vi "Tosca-Init Data File.vi"(0 "Path":path, 5 "Tosca":refnum<class "Parameters.lvclass">, 11 "error in (no error)":errorcluster) -> (15 "error out":errorcluster)   [LabVIEW 2020]
uses:
  Classes/Parameters/Parameters.lvclass
  Classes/Parameters/Parameters.lvclass/Parameters.ctl
  Classes/Parameters/Read ParamFile.vi
  Classes/Parameters/Read Pretrial.vi
  Tosca-Globals.vi
panel:
  in  "Info":T1
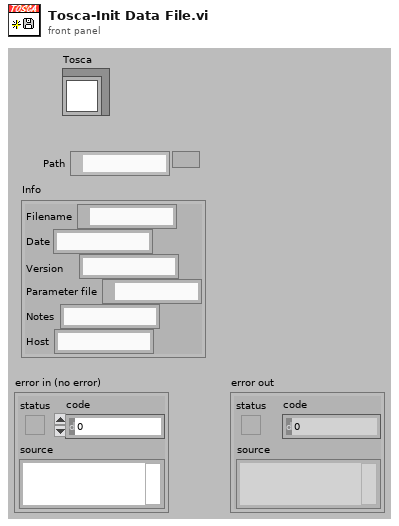
[diagram p1: front panel]
types:
  T1 = cluster{"Filename":path, "Date":string, "Version":string, "Parameter file":path, "Notes":string, "Host":string}
  T2 = typedef "Tosca-Pretrial Spec.ctl" = cluster{"Path":path, "Args":string[]}
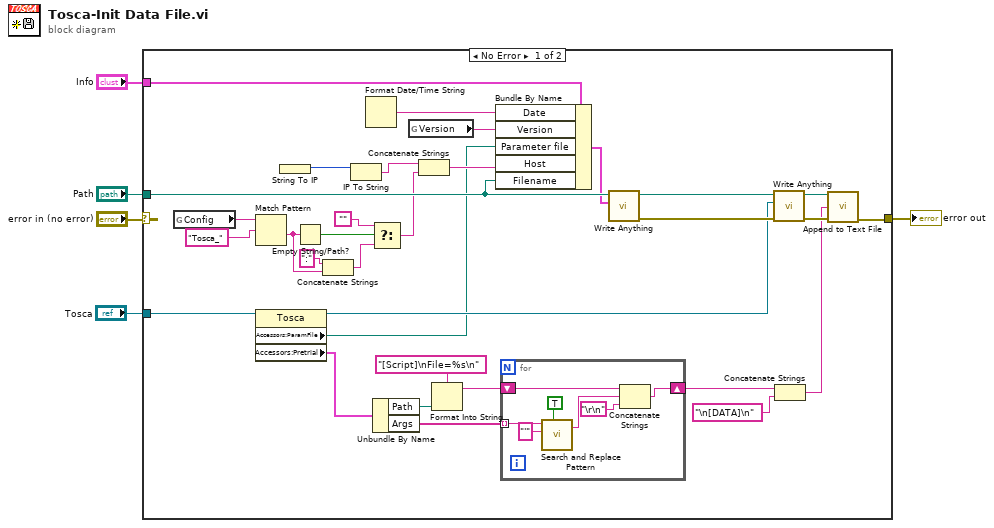
[diagram p0: block diagram]
diagram:
  n1 = case shown="No Error" "error in (no error)" {
    selector: "error in (no error)" -> [_ w45]
    tunnel: [w29 w45] -> w4
    tunnel: "Info" -> [w36 _]
    tunnel: "Path" -> [w35 _]
    tunnel: "Tosca" -> [w16 _]
    frame No Error {
      n2 = global read "Tosca-Globals.vi" "Config"() -> (w25:string)
      n3 = Match Pattern(string=w25, regular expression="Tosca_") -> (after substring=w20:string)  [unwired: 1 in, 3 out]
      n4 = property class="Tosca"(reference=w16) -> (reference out=w9:refnum<class "Parameters.lvclass">, "Accessors:ParamFile"=w7:path, "Accessors:Pretrial"=w8:T2)  [unwired: 1 in, 1 out]
      n5 = String To IP() -> (0:w27:u32)  [unwired: 1 in]
      n6 = Empty String/Path?(string/path=w20) -> (empty?=w22:bool)
      n7 = Concatenate Strings(":" ("string"), w20) -> (w18:string)
      n8 = IP To String(2:w27) -> (0:w26:string)  [unwired: 1 in]
      n9 = Format Date/Time String() -> (date/time string=w37:string)  [unwired: 3 in]
      n10 = Select(t="", s=w22, f=w18) -> (s? t:f=w21:string)
      n11 = Unbundle By Name(w8) -> ("Path"=w14:path, "Args"=w13:string[])
      n12 = global read "Tosca-Globals.vi" "Version"() -> (w6:string)
      n13 = Concatenate Strings(w26, w21) -> (w23:string)
      n14 = Format Into String(format string="[Script]\nFile=%s\n", w14) -> (resulting string=w12:string)  [unwired: 2 in, 1 out]
      n15 = Bundle By Name(cluster=w36, "Date"=w37, "Version"=w6, "Parameter file"=w7, "Host"=w23, "Filename"=w35) -> (w34:T1)
      n16 = for {
        tunnel: w13 -> [w40] mode=indexing
        shift-right: [w43] -> w11
        shift-left: w12 -> [w44]
        n17 = call <vilib>:"Search and Replace Pattern.vi"("string"=w40, "regular expression (\"\")"="'" ("regular expression (\"\")"), "replace all? (F)"=TRUE) -> ("result string"=w41:string)  [unwired: 2 in, 1 out]
        n18 = Concatenate Strings(w44, w41, "\r\n") -> (w43:string)
      }
      n19 = call "Write Anything.vi"("Anything"=w34, "Path (dialog)"=w35) -> ("Error Out"=w33:errorcluster, "Path out"=w32:path)  [unwired: 8 in]
      n20 = call "Write Anything.vi"("Error In"=w33, "Anything"=w9, "Path (dialog)"=w32) -> ("Error Out"=w31:errorcluster, "Path out"=w30:path)  [unwired: 7 in]
      n21 = Concatenate Strings(w11, "\n[DATA]\n" ("Section Name (Name of \"Anything\")")) -> (w28:string)
      n22 = call "Append to Text File.vi"("file path"=w30, "text"=w28, "error in (no error)"=w31) -> ("error out"=w29:errorcluster)  [unwired: 11 in, 1 out]
    }
    frame Error {
    }
  }
  "error out" <- w4
